vi "PH_BL-Master.Find Boolean GUI Ref by Name.vi"(2 "Boolean Ref Array":refnum<vi>[](array[refnum]), 4 "Label":string, 5 "error in (no error)":errorcluster) -> (16 "Wanted Boolean Ref":refnum<vi>, 17 "index of element":i32, 18 "Ref found?":bool, 19 "error out":errorcluster)   [LabVIEW 2014, in "PH_BL-Master.lvlib"]
doc: "By this VI a GUI reference of a boolean GUI element is found from a reference array by its label name."
uses:
  PH_BL-Master.lvlib
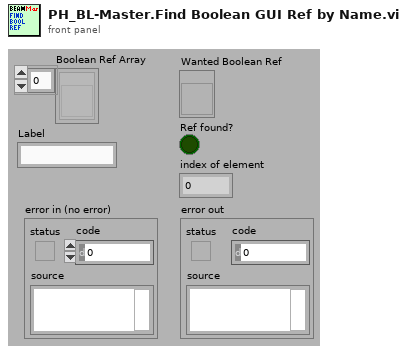
[diagram p1: front panel]
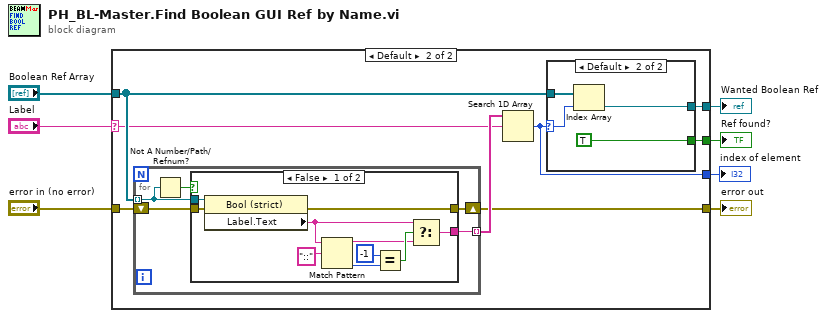
[diagram p0: block diagram]
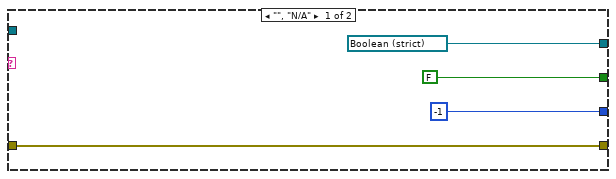
[diagram p2: hidden frame]
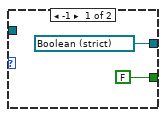
[diagram p3: hidden frame]
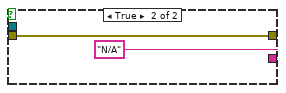
[diagram p4: hidden frame]
diagram:
  n1 = case shown="Default" "Label" {
    selector: "Label" -> [_ w12]
    tunnel: "Boolean Ref Array" -> [_ w18]
    tunnel: [refnum<vi> refnum ("6P") w17] -> w6
    tunnel: [w8 w16] -> w5
    tunnel: "error in (no error)" -> [w8 w15]
    tunnel: [-1 ("index of element") w14] -> w3
    tunnel: [FALSE w13] -> w2
    frame "", "N/A" {
    }
    frame Default {
      n2 = for {
        tunnel: w18 -> [w26] mode=indexing
        tunnel: [w30] -> w19 mode=indexing
        shift-right: [w29] -> w16
        shift-left: w15 -> [w28]
        n3 = Not A Number/Path/Refnum?(number/path/refnum=w26) -> (NaN/Path/Refnum?=w27:bool)
        n4 = case shown="False" w27 {
          tunnel: w26 -> [w40 _]
          tunnel: [w34 "N/A" ("Label.Text")] -> w30
          tunnel: [w39 w41] -> w29
          tunnel: w28 -> [w38 w41]
          frame False {
            n5 = property class="Bool (strict)"(reference=w40, error in=w38) -> (error out=w39:errorcluster, "Label.Text"=w35:string)  [unwired: 1 out]
            n6 = Match Pattern(string=w35, regular expression="::") -> (before substring=w33:string, offset past match=w32:i32)  [unwired: 1 in, 2 out]
            n7 = Equal?(x=-1 ("y"), y=w32) -> (x = y?=w36:bool)
            n8 = Select(t=w35, s=w36, f=w33) -> (s? t:f=w34:string)
          }
          frame True {
          }
        }
      }
      n9 = Search 1D Array(1D array=w19, element=w12) -> (index of element=w14:i32)  [unwired: 1 in]
      n10 = case shown="Default" w14 {
        selector: w14 -> [_ w23]
        tunnel: w18 -> [_ w25]
        tunnel: [refnum<vi> refnum ("6P") w24] -> w17
        tunnel: [FALSE TRUE] -> w13
        frame -1 {
        }
        frame Default {
          n11 = Index Array(array=w25, index=w23) -> (element=w24:refnum<vi>)
        }
      }
    }
  }
  "Wanted Boolean Ref" <- w6
  "error out" <- w5
  "Ref found?" <- w2
  "index of element" <- w3
